vi "Read DAQ Class.lvclass.vi"(8 "error in (no error)":errorcluster, 11 "Processing in":refnum<class "Processing.lvclass">) -> (0 "error out":errorcluster, 2 "DAQ Class.lvclass":refnum<class "DAQ Class.lvclass">, 3 "Processing out":refnum<class "Processing.lvclass">)   [LabVIEW 2014, in "Processing.lvclass"]
uses:
  Processing.lvclass
  DAQ/DAQ Class.lvclass
  Processing.lvclass/Processing.ctl
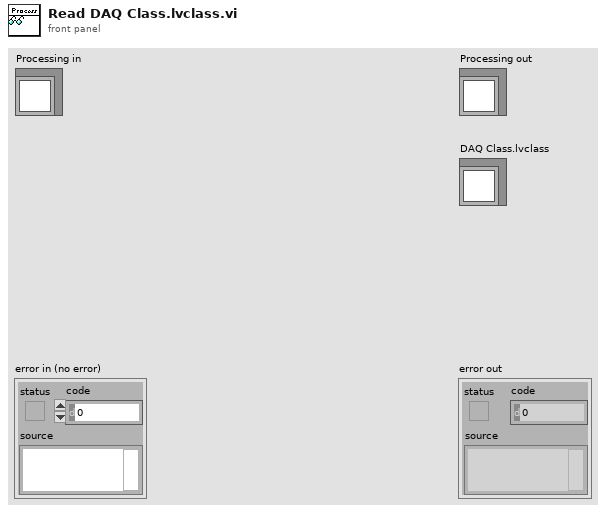
[diagram p1: front panel]
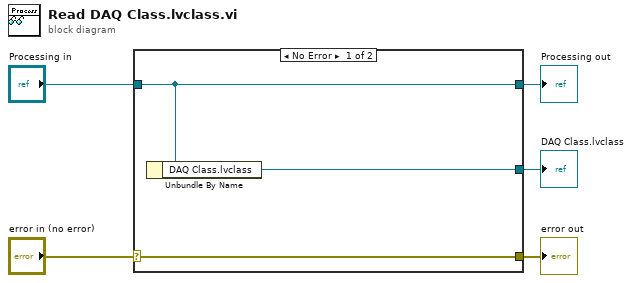
[diagram p0: block diagram]
diagram:
  n1 = case shown="No Error" "error in (no error)" {
    selector: "error in (no error)" -> [w8 w9]
    tunnel: [w8 w9] -> w4
    tunnel: [w7 w10] -> w2
    tunnel: "Processing in" -> [w7 w10]
    tunnel: [w6 _] -> w1
    frame No Error {
      n2 = Unbundle By Name(w7) -> ("DAQ Class.lvclass"=w6:refnum<class "DAQ Class.lvclass">)
    }
    frame Error {
    }
  }
  "error out" <- w4
  "Processing out" <- w2
  "DAQ Class.lvclass" <- w1
